vi "DataVIS_Differentiate_and_Rebundle.vi"(7 "Fit Points":dbl, 8 "error in (no error)":errorcluster, 10 "IV":cluster{dbl[], dbl[]}[][][](array[cluster]), 11 "IV-2T":cluster{dbl[], dbl[]}[][][](array[cluster])) -> (0 "error out":errorcluster, 3 "Data Cell":T1(array[cluster]))   [LabVIEW 2016]
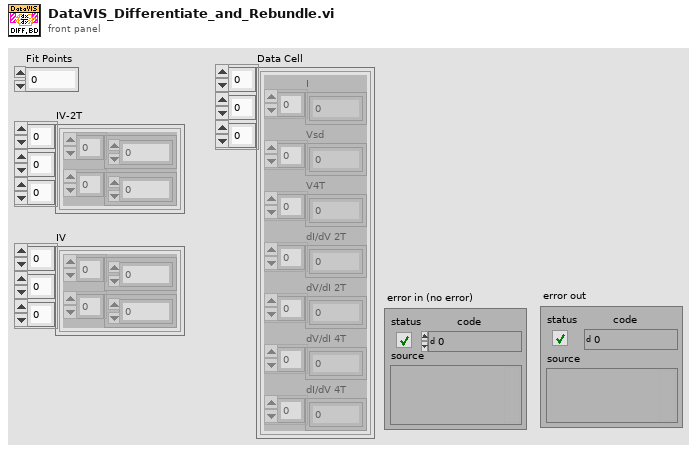
[diagram p1: front panel]
types:
  T1 = cluster{"I":dbl[], "Vsd":dbl[], "V4T":dbl[], "dI/dV 2T":dbl[], "dV/dI 2T":dbl[], "dV/dI 4T":dbl[], "dI/dV 4T":dbl[]}[][][]
  T2 = cluster{"I":dbl[], "Vsd":dbl[], "V4T":dbl[], "dI/dV 2T":dbl[], "dV/dI 2T":dbl[], "dV/dI 4T":dbl[], "dI/dV 4T":dbl[]}
  T3 = cluster{"Decimated Array":dbl[], "Decimated Array":dbl[]}
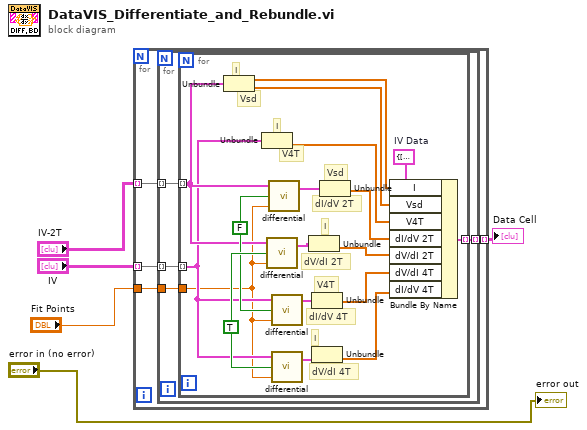
[diagram p0: block diagram]
diagram:
  n1 = for {
    tunnel: "IV" -> [w9] mode=indexing
    tunnel: "IV-2T" -> [w8] mode=indexing
    tunnel: [w7] -> w4 mode=indexing
    tunnel: "Fit Points" -> [w6]
    n2 = for {
      tunnel: w9 -> [w13] mode=indexing
      tunnel: w8 -> [w12] mode=indexing
      tunnel: [w11] -> w7 mode=indexing
      tunnel: w6 -> [w10]
      n3 = for {
        tunnel: w13 -> [w24] mode=indexing
        tunnel: w12 -> [w25] mode=indexing
        tunnel: [w15] -> w11 mode=indexing
        tunnel: w10 -> [w14]
        w23 = T2 {"I"=[], "Vsd"=[], "V4T"=[], "dI/dV 2T"=[], "dV/dI 2T"=[], "dV/dI 4T"=[], "dI/dV 4T"=[]}  # IV Data
        w30 = FALSE ("dy/dx vs x")
        w31 = TRUE ("dy/dx vs x")
        # "V4T"
        # "I"
        # "Vsd"
        # "I"
        # "dV/dI 4T"
        # "I"
        # "dI/dV 4T"
        # "V4T"
        # "dV/dI 2T"
        # "I"
        # "dI/dV 2T"
        # "Vsd"
        n4 = Unbundle(w25) -> (w22:dbl[], w21:dbl[])
        n5 = Unbundle(w24) -> (w20:dbl[])  [unwired: 1 out]
        n6 = call <userlib>:"differential.vi"("Numeric"=w14, "dy/dx vs x"=w31, "A vs B 2"=w25) -> ("A vs B 3"=w26:T3)  [unwired: 1 in]
        n7 = call <userlib>:"differential.vi"("Numeric"=w14, "dy/dx vs x"=w30, "A vs B 2"=w25) -> ("A vs B 3"=w29:T3)  [unwired: 1 in]
        n8 = call <userlib>:"differential.vi"("Numeric"=w14, "dy/dx vs x"=w30, "A vs B 2"=w24) -> ("A vs B 3"=w27:T3)  [unwired: 1 in]
        n9 = call <userlib>:"differential.vi"("Numeric"=w14, "dy/dx vs x"=w31, "A vs B 2"=w24) -> ("A vs B 3"=w28:T3)  [unwired: 1 in]
        n10 = Unbundle(w26) -> ("Decimated Array"=w18:dbl[])  [unwired: 1 out]
        n11 = Unbundle(w27) -> ("Decimated Array"=w17:dbl[])  [unwired: 1 out]
        n12 = Unbundle(w28) -> ("Decimated Array"=w16:dbl[])  [unwired: 1 out]
        n13 = Unbundle(w29) -> ("Decimated Array"=w19:dbl[])  [unwired: 1 out]
        n14 = Bundle By Name(cluster=w23, "I"=w22, "Vsd"=w21, "V4T"=w20, "dI/dV 2T"=w19, "dV/dI 2T"=w18, "dV/dI 4T"=w17, "dI/dV 4T"=w16) -> (w15:T2)
      }
    }
  }
  "Data Cell" <- w4
  "error out" <- "error in (no error)"
